vi "TWM Client Cmd Get Result.vi"(4 "phase ref channel tag (none)":string, 5 "timeout [s] (10s)":dbl=10.0, 6 "qwtb maxdim (scalar)":T3 caption="Max. shown dimension (scalar)", 7 "end of packet key":string="TWM:command:EndOfPacket", 8 "error in":errorcluster, 9 "quantity names (all)":string[](array[string]), 10 "meas root path (last)":path, 11 "handle":i32) -> (0 "error out":errorcluster, 1 "result info":T1, 2 "result data":T2[][](array[typedef]), 3 "handle out":i32)   [LabVIEW 2013, in "TWM Client.lvlib"]
doc: "Write Get result command packet to TWM server. Get answer. Set reasonable timeout for the TWM processing, because it has to load, process and format the result before sending."
uses:
  TWM Client.lvlib
  TWM Client Result Max Dim.ctl
  TWM Client Quantity Record.ctl
  TWM Client Result Info.ctl
  octave/infolib.lvlibp/Private/Add key polymorph parts/String.vi
  octave/infolib.lvlibp/Private/Add matrix polymorph parts/1D String.vi
  octave/infolib.lvlibp/Private/Add key polymorph parts/I64.vi
  octave/infolib.lvlibp/Private/Add key polymorph parts/EXT.vi
  octave/infolib.lvlibp/Private/Get matrix polymorph parts/Get 1D String.vi
  octave/infolib.lvlibp/Private/Get key polymorph parts/GetI64.vi
  octave/infolib.lvlibp/Private/Get key polymorph parts/GetString.vi
  <vilib>/Utility/error.llb/Error Cluster From Error Code.vi
  octave/infolib.lvlibp/Private/Get matrix polymorph parts/Get 1D EXT.vi
  <vilib>/ErrorRing/Error Ring.xnode
  octave/infolib.lvlibp
panel:
  out "result info":T1
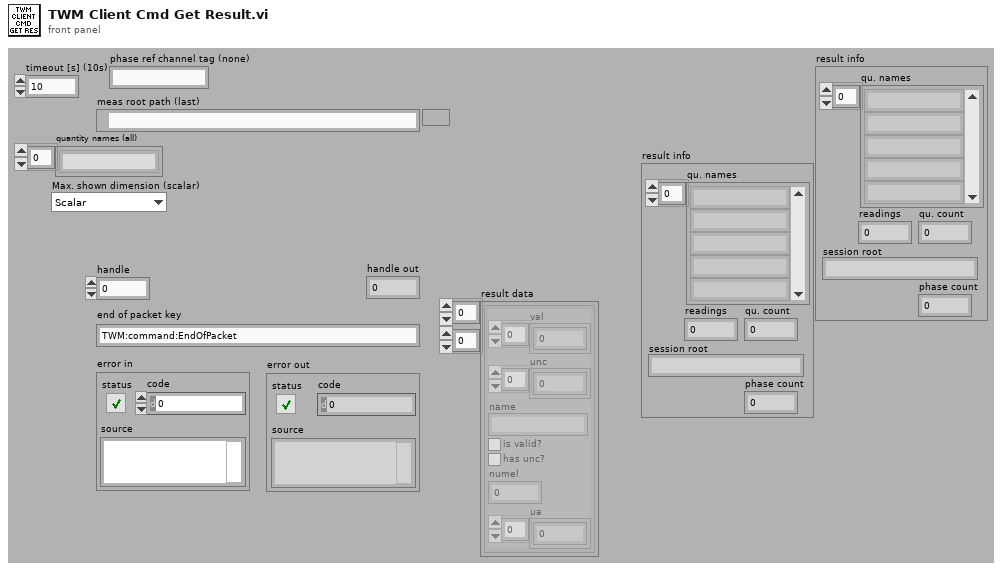
[diagram p1: front panel]
types:
  T1 = typedef "TWM Client.lvlib/TWM Client Result Info.ctl" = cluster{"qu. names":string[], "readings":i32, "qu. count":i32, "session root":string, "phase count":i32}
  T2 = typedef "TWM Client.lvlib/TWM Client Quantity Record.ctl" = cluster{"val":dbl[], "unc":dbl[], "name":string, "is valid?":bool, "has unc?":bool, "numel":i32, "ua":dbl[]}
  T3 = typedef "TWM Client.lvlib/TWM Client Result Max Dim.ctl" = enum16{"Scalar", "Vector", "Matrix"}
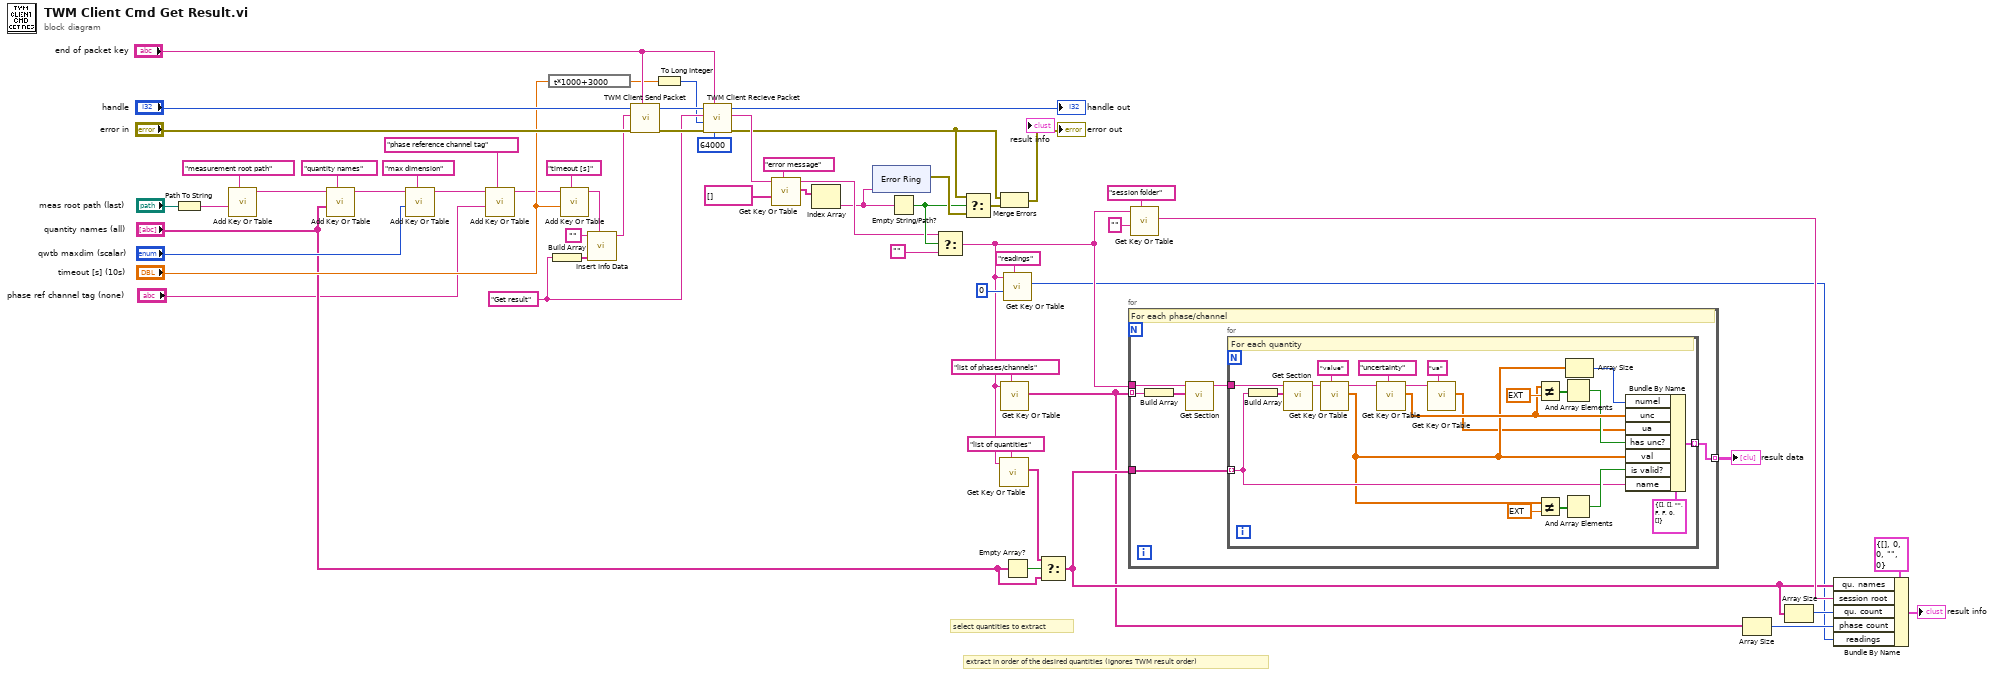
[diagram p0: block diagram]
diagram:
  w40 = "Get result" ("key string")
  # "extract in order of the desired quantities (ignores TWM result order)"
  # "select quantities to extract"
  n1 = Path To String(path="meas root path (last)") -> (string=w48:string)
  n2 = call-poly "Add Key Or Table.vi"("key description"="measurement root path", "string"=w48) -> ("info data out"=w51:string)  [unwired: 8 in, 1 out]
  n3 = call-poly "Add Key Or Table.vi"("key description"="quantity names", "string"="quantity names (all)", "info data"=w51) -> ("info data out"=w46:string)  [unwired: 7 in, 1 out]
  n4 = call-poly "Add Key Or Table.vi"("key description"="max dimension", "numeric"="qwtb maxdim (scalar)", "info data"=w46) -> ("info data out"=w20:string)  [unwired: 7 in, 1 out]
  n5 = call-poly "Add Key Or Table.vi"("key description"="phase reference channel tag", "string"="phase ref channel tag (none)", "info data"=w20) -> ("info data out"=w19:string)  [unwired: 7 in, 1 out]
  n6 = expression code="t*1000+3000"("timeout [s] (10s)") -> (w34:dbl)
  n7 = Build Array(w40) -> (w41:string[])
  n8 = call-poly "Add Key Or Table.vi"("key description"="timeout [s]", "numeric"="timeout [s] (10s)", "info data"=w19) -> ("info data out"=w42:string)  [unwired: 7 in, 1 out]
  n9 = call "Insert Info Data.vi"("info data to insert"=w42, "sections"=w41, "info data"="") -> ("info data out"=w38:string)  [unwired: 7 in, 1 out]
  n10 = call "TWM Client Send Packet.vi"("end of packet key"="end of packet key", "error in"="error in", "command string"=w38, "handle"="handle") -> ("error out"=w57:errorcluster, "handle out"=w55:i32)  [unwired: 6 in]
  n11 = To Long Integer(number=w34) -> (32bit integer=w33:i32)
  n12 = call "TWM Client Recieve Packet.vi"("max message length (1024)"=64000, "end of packet key"="end of packet key", "error in"=w57, "timeout [ms] (5000 ms)"=w33, "message header (empty)"=w40, "handle in"=w55) -> ("error out"=w30:errorcluster, "message data"=w52:string, "handle out"=→"handle out":i32)  [unwired: 3 in]
  n13 = call-poly "Get Key Or Table.vi"("key description"="error message", "string"=string[] [], "info data"=w52) -> ("value"=w31:string[], "info data out"=w27:string)  [unwired: 5 in, 2 out]
  n14 = Index Array(array=w31) -> (element=w15:string)  [unwired: 1 in]
  n15 = xnode "Error Ring"("parameter 0"=w15) -> ("error out"=w29:errorcluster)
  n16 = Empty String/Path?(string/path=w15) -> (empty?=w28:bool)
  n17 = Select(t=w27, s=w28, f="") -> (s? t:f=w10:string)
  n18 = Select(t=w30, s=w28, f=w29) -> (s? t:f=w37:errorcluster)
  n19 = call-poly "Get Key Or Table.vi"("key description"="list of quantities", "info data"=w10) -> ("value"=w21:string[])  [unwired: 6 in, 3 out]
  n20 = Merge Errors(w30, w37) -> (→"error out":errorcluster)
  n21 = call-poly "Get Key Or Table.vi"("key description"="list of phases/channels", "info data"=w10) -> ("value"=w3:string[])  [unwired: 6 in, 3 out]
  n22 = call-poly "Get Key Or Table.vi"("key description"="readings", "numeric"=i64 0, "info data"=w10) -> ("value"=w2:i64)  [unwired: 5 in, 3 out]
  n23 = Empty Array?(array="quantity names (all)") -> (empty?=w23:bool)
  n24 = Select(t=w21, s=w23, f="quantity names (all)") -> (s? t:f=w5:string[])
  n25 = for {
    tunnel: w3 -> [w64] mode=indexing
    tunnel: w10 -> [w65]
    tunnel: w5 -> [w60]
    tunnel: [w61] -> w24 mode=indexing
    # "For each phase/channel"
    n26 = Build Array(w64) -> (w63:string[])
    n27 = call "Get Section.vi"("sections"=w63, "info data"=w65) -> ("section part"=w62:string)  [unwired: 8 in, 1 out]
    n28 = for {
      tunnel: w62 -> [w86]
      tunnel: [w72] -> w61 mode=indexing
      tunnel: w60 -> [w71] mode=indexing
      # "For each quantity"
      n29 = Build Array(w71) -> (w85:string[])
      n30 = call "Get Section.vi"("sections"=w85, "info data"=w86) -> ("section part"=w83:string)  [unwired: 8 in, 1 out]
      n31 = call-poly "Get Key Or Table.vi"("key description"="value", "info data"=w83) -> ("value"=w70:ext[], "info data out"=w80:string)  [unwired: 6 in, 2 out]
      n32 = call-poly "Get Key Or Table.vi"("key description"="uncertainty", "info data"=w80) -> ("value"=w74:ext[], "info data out"=w67:string)  [unwired: 6 in, 2 out]
      n33 = call-poly "Get Key Or Table.vi"("key description"="ua", "info data"=w67) -> ("value"=w66:ext[])  [unwired: 6 in, 3 out]
      n34 = Not Equal?(x=w74, y=ext nan) -> (x != y?=w76:bool[])
      n35 = Not Equal?(x=w70, y=ext nan) -> (x != y?=w78:bool[])
      n36 = And Array Elements(Boolean array=w76) -> (logical AND=w73:bool)
      n37 = And Array Elements(Boolean array=w78) -> (logical AND=w77:bool)
      n38 = Array Size(array=w70) -> (size(s)=w69:i32)
      n39 = Bundle By Name(cluster=T2 {"val"=[], "unc"=[], "name"="", "is valid?"=FALSE, "has unc?"=FALSE, "numel"=0, "ua"=[]} ("quantity"), "numel"=w69, "unc"=w74, "ua"=w66, "has unc?"=w73, "val"=w70, "is valid?"=w77, "name"=w71) -> (w72:T2)
    }
  }
  "result data" <- w24
  n40 = call-poly "Get Key Or Table.vi"("key description"="session folder", "string"="", "info data"=w10) -> ("value"=w7:string)  [unwired: 5 in, 3 out]
  n41 = Array Size(array=w3) -> (size(s)=w4:i32)
  n42 = Array Size(array=w5) -> (size(s)=w6:i32)
  n43 = Bundle By Name(cluster=T1 {"qu. names"=[], "readings"=0, "qu. count"=0, "session root"="", "phase count"=0} ("result info"), "qu. names"=w5, "session root"=w7, "qu. count"=w6, "phase count"=w4, "readings"=w2) -> (→"result info":T1)
